vi "Read BBM.vi"(8 "error in (no error)":errorcluster, 11 "WorkTable Class in":refnum<class "WorkTable Class.lvclass">) -> (0 "error out":errorcluster, 2 "BBM":T3, 3 "WorkTable Class out":refnum<class "WorkTable Class.lvclass">)   [LabVIEW 2011, in "WorkTable Class.lvclass"]
uses:
  WorkTable Class.lvclass
  Type Definitions/Worktable_BBM Slot.ctl
  Vec3d Class/Vec3d Class.lvclass
  Orient3d Class/Orient3d Class.lvclass
  Utils/Type Definitions/Position_Orientation.ctl
  WorkTable Class.lvclass/WorkTable Class.ctl
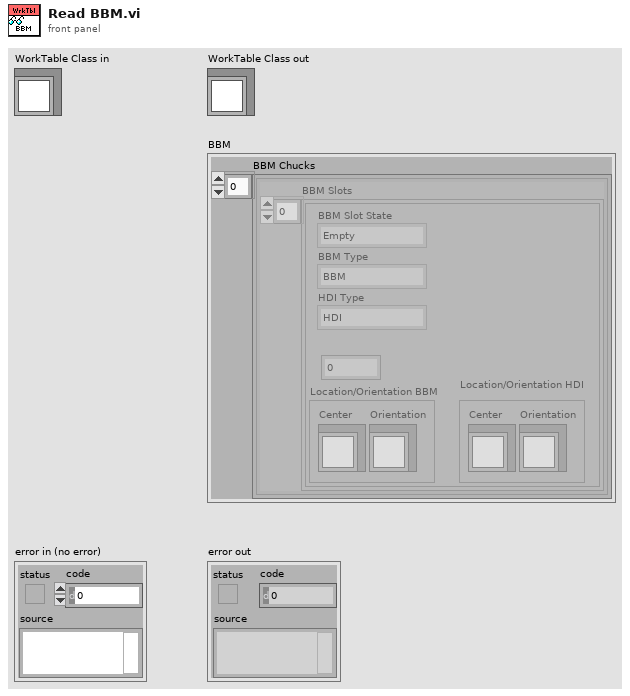
[diagram p1: front panel]
types:
  T1 = typedef "Worktable_BBM Slot.ctl" = cluster{"BBM Slot State":enum16{"Empty", "Unglued", "Stamped", "PartOnTop", "Weighted", "Unpotted", "Potted"}, "BBM Type":enum16{"BBM", "GlassSlide"}, "HDI Type":enum16{"HDI", "Polyimide"}, "Vacuum Channel":u8, "Location/Orientation BBM":T2, "Location/Orientation HDI":T2}
  T2 = typedef "Position_Orientation.ctl" = cluster{"Center":refnum<class "Vec3d Class.lvclass">, "Orientation":refnum<class "Orient3d Class.lvclass">}
  T3 = cluster{"BBM Chucks":cluster{"BBM Slots":T1[]}[]}
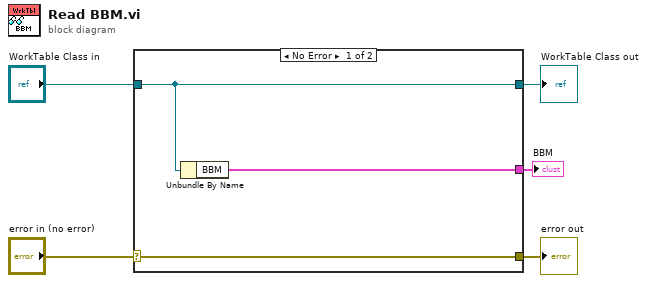
[diagram p0: block diagram]
diagram:
  n1 = case shown="No Error" "error in (no error)" {
    selector: "error in (no error)" -> [w8 w9]
    tunnel: [w8 w9] -> w4
    tunnel: [w7 w10] -> w2
    tunnel: "WorkTable Class in" -> [w7 w10]
    tunnel: [w6 _] -> w1
    frame No Error {
      n2 = Unbundle By Name(w7) -> ("BBM"=w6:T3)
    }
    frame Error {
    }
  }
  "error out" <- w4
  "WorkTable Class out" <- w2
  "BBM" <- w1
